vi "ADS_MUX.vi"(1 "Board address":i32=4660 format="%x", 2 "error in (no error)":errorcluster, 3 "In Neg":enum16{"OPEN", "GND", "DAC", "No Change"}(ring), 4 "In Pos":enum16{"OPEN", "GND", "DAC", "No Change"}(ring), 5 "Mux Num":enum16{"ADS1", "ADS2"}(ring)) -> (0 "error out":errorcluster)   [LabVIEW 2011]
doc: "This VI sets the USB-DAQ analog debug multiplexer. The Mux allows the DAC to be connected to the ADC for debug / calibration. Normally the inputs can be left disconnected (OPEN). This can be called once at the start of the program if you do not need to use this debug feature."
panel:
  # "Inputs"
  # "Outputs"
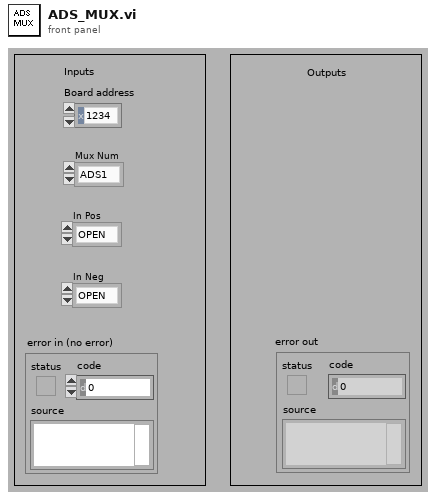
[diagram p1: front panel]
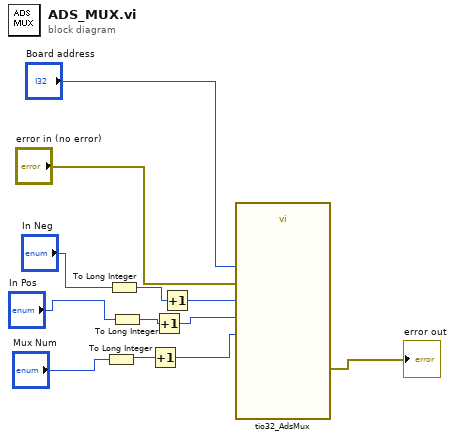
[diagram p0: block diagram]
diagram:
  n1 = To Long Integer(number="Mux Num") -> (32bit integer=w6:i32)
  n2 = To Long Integer(number="In Neg") -> (32bit integer=w1:i32)
  n3 = To Long Integer(number="In Pos") -> (32bit integer=w3:i32)
  n4 = Increment(x=w6) -> (x+1=w5:i32)
  n5 = Increment(x=w3) -> (x+1=w4:i32)
  n6 = Increment(x=w1) -> (x+1=w2:i32)
  n7 = call "tio32_AdsMux.vi"("Board address"="Board address", "MUX number"=w5, "error in (no error)"="error in (no error)", "Input P"=w4, "Input N"=w2) -> ("error out"=→"error out":errorcluster)  [unwired: 8 in, 2 out]
